vi "CreatePrivateEvents.vi"(8 "error in (no error)":errorcluster, 11 "XYStage":refnum<class "XYStage.lvclass">) -> (0 "error out":errorcluster, 3 "XYStage out":refnum<class "XYStage.lvclass">)   [LabVIEW 2017, in "XYStage.lvclass"]
doc: "---------------------------------------------------------------\nJKI State Machine Objects™\nhttp://jki.net/state-machine-objects/\nCopyright (C) 2005-2015, JKI <info@jki.net>\nALL RIGHTS RESERVEDJKI State Machine Objects (SMO) 1.0.0.4\nJKI - JKI\nCopyright (c) 2015, JKI"
uses:
  XYStage.lvclass
  XYStage.lvclass/XYStage.ctl
  Typedefs/PrivateEvents--XYStage.MoveAbsolute (units).ctl
  Typedefs/Coordinates.Units--Cluster.ctl
  Device/Device.lvclass
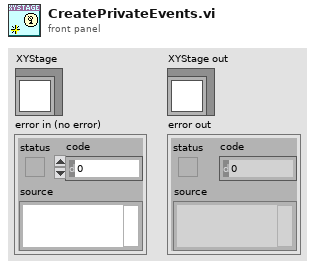
[diagram p1: front panel]
types:
  T1 = typedef "XYStage.lvclass/PrivateData--Ref.ctl" = refnum<data-value>
  T2 = typedef "XYStage.lvclass/PrivateEvents--XYStage.MoveAbsolute (units).ctl" = cluster{"Coordinates.Units":T3, "Wait Timeout, ms":i32}
  T3 = typedef "XYStage.lvclass/Coordinates.Units--Cluster.ctl" = cluster{"X":dbl, "Y":dbl}
  T4 = typedef "XYStage.lvclass/PrivateData--Cluster.ctl" = cluster{"Configuration":T5, "Public Events":T6, "Protected Events":T7, "Private Events":T8}
  T5 = typedef "XYStage.lvclass/Configuration--Cluster.ctl" = cluster{"Serial Number":string, "X Axis":string, "Y Axis":string, "Real-World Units":string, "Counts per Unit":u32}
  T6 = typedef "XYStage.lvclass/PublicEvents--Cluster.ctl" = cluster{"MoveStarted":refnum<user-event>, "MoveCompleted":refnum<user-event>}
  T7 = typedef "XYStage.lvclass/ProtectedEvents--Cluster.ctl" = cluster{"StatusUpdated":refnum<user-event>}
  T8 = typedef "XYStage.lvclass/PrivateEvents--Cluster.ctl" = cluster{"MoveAbsolute (units)":refnum<user-event>}
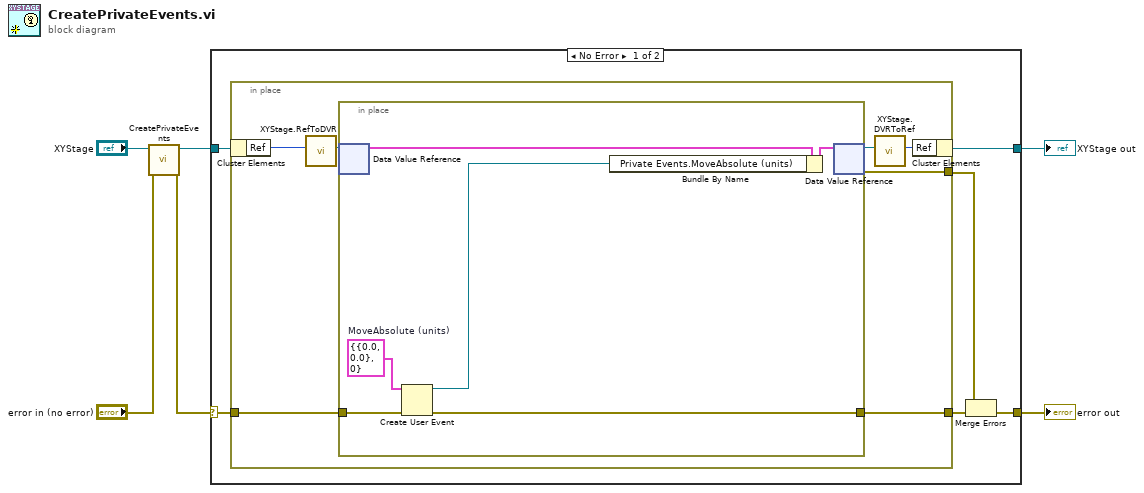
[diagram p0: block diagram]
diagram:
  n1 = call-parent "CreatePrivateEvents.vi"("error in (no error)"="error in (no error)", "SMO"="XYStage") -> ("error out"=w1:errorcluster, "SMO out"=w3:refnum<class "XYStage.lvclass">)  [unwired: 8 in]
  n2 = case shown="No Error" w1 {
    selector: w1 -> [w10 w27]
    tunnel: [w8 w27] -> w5
    tunnel: [w11 w26] -> w6
    tunnel: w3 -> [w12 w26]
    frame No Error {
      n3 = in-place {
        in-place-border: w10 -> [w19]
        in-place-border: [w16] -> w7
        in-place-border: [w15] -> w9
        n4 = in-place-cluster #1(w12) -> ("Ref"=w18:u32)
        n5 = call "XYStage.RefToDVR.vi"("Ref"=w18) -> ("Ref"=w14:T1)  [unwired: 10 in]
        n6 = in-place {
          in-place-border: w19 -> [w25]
          in-place-border: [w22] -> w16
          w20 = T2 {"Coordinates.Units"={"X"=0.0, "Y"=0.0}, "Wait Timeout, ms"=0}  # MoveAbsolute (units)
          n7 = in-place-dvr #2(w14) -> (w24:T4)  [unwired: 1 out]
          n8 = Create User Event(user event datatype=w20, error in=w25) -> (user event=w21:refnum<user-event>, error out=w22:errorcluster)
          n9 = Bundle By Name(cluster=w24, "Private Events.MoveAbsolute (units)"=w21) -> (w23:T4)
          n10 = in-place-dvr #2(w23) -> (w17:T1, w15:errorcluster)
        }
        n11 = call "XYStage.DVRToRef.vi"("Ref"=w17) -> ("Ref"=w13:u32)  [unwired: 10 in]
        n12 = in-place-cluster #1("Ref"=w13) -> (w11:refnum<class "XYStage.lvclass">)
      }
      n13 = Merge Errors(w9, w7) -> (w8:errorcluster)
    }
    frame Error {
    }
  }
  "error out" <- w5
  "XYStage out" <- w6
